vi "RemoveHandler.vi"(0 "Config in":T1, 5 "Server Index":i32, 7 "HandlerName":string, 11 "error in (no error)":errorcluster) -> (4 "Config out":T1, 15 "error out":errorcluster)   [LabVIEW 2017]
uses:
  <vilib>/WebServerConfig/Config.ctl
  <vilib>/WebServerConfig/Server.ctl
  <vilib>/WebServerConfig/Alias.ctl
  <vilib>/WebServerConfig/ErrorDocument.ctl
  <vilib>/WebServerConfig/Action.ctl
  <vilib>/WebServerConfig/Redirect.ctl
  <vilib>/WebServerConfig/Interface.ctl
  <vilib>/WebServerConfig/AddHandler.ctl
  <vilib>/WebServerConfig/SSL.ctl
  <vilib>/WebServerConfig/CustomLog.ctl
  <vilib>/WebServerConfig/LoadModule.ctl
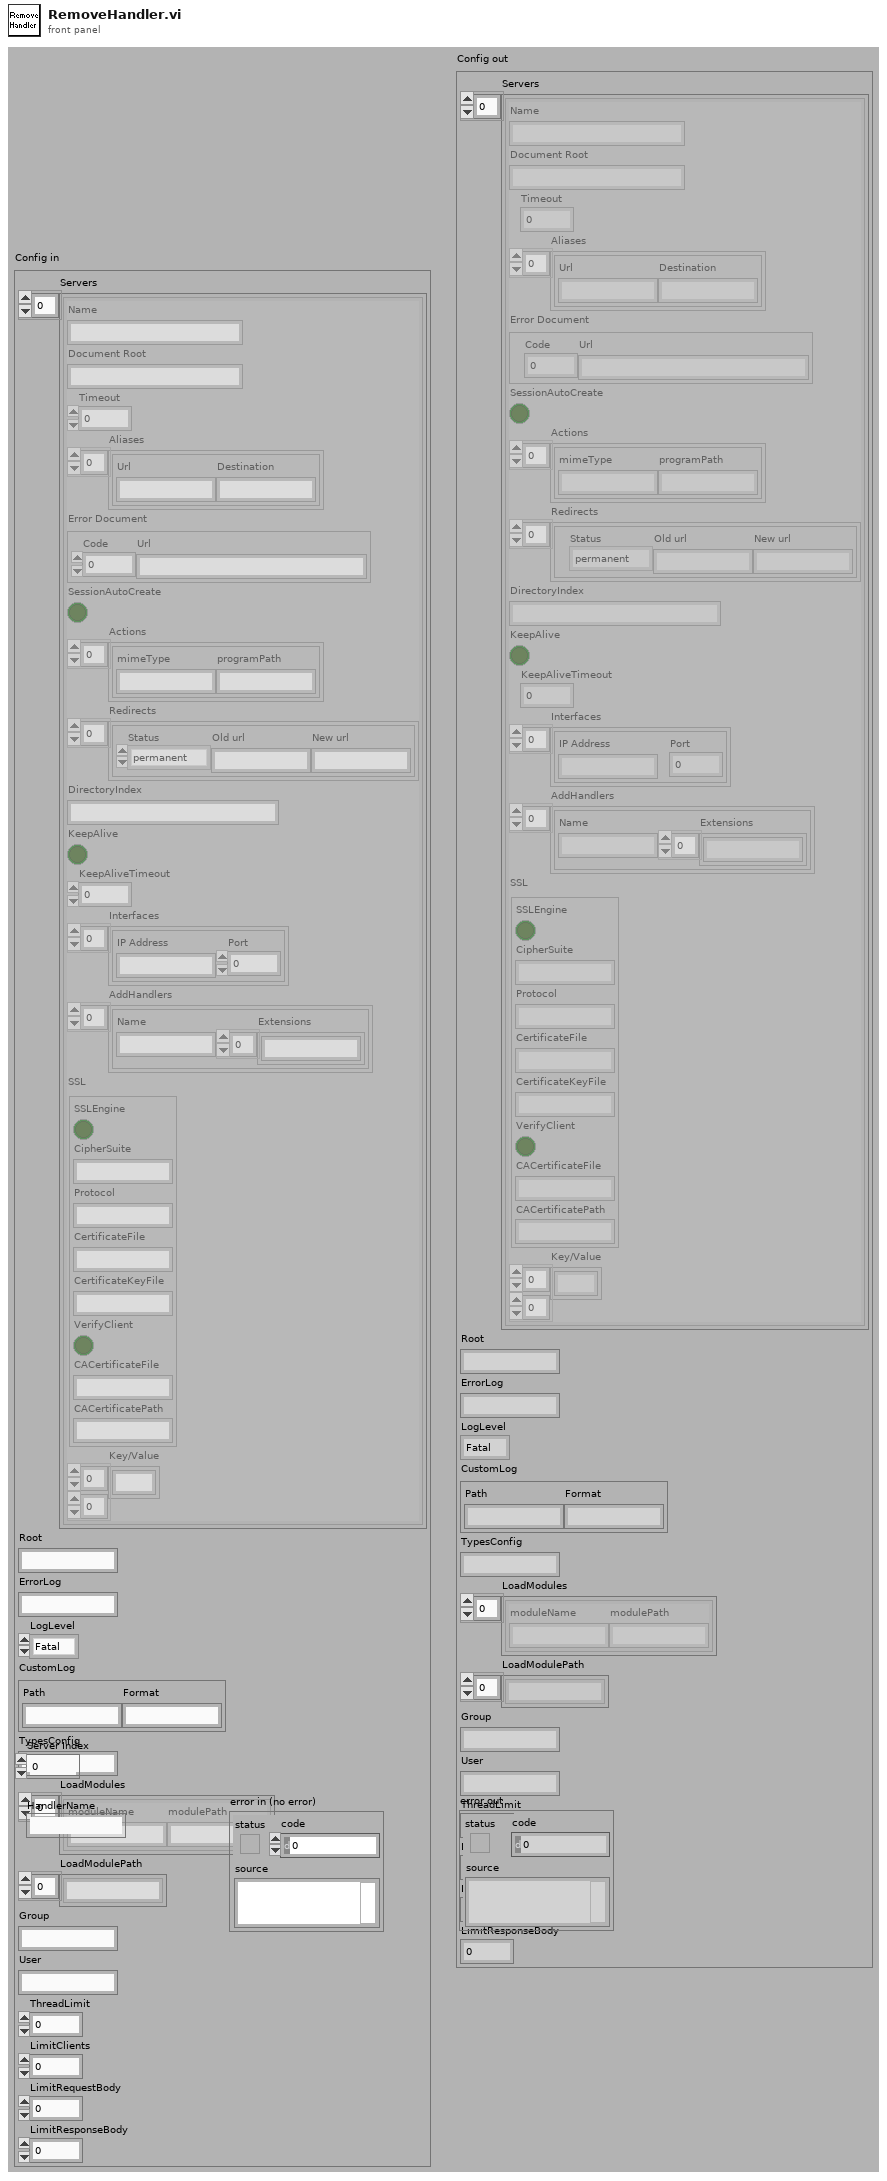
[diagram p1: front panel]
types:
  T1 = typedef "Config.ctl" = cluster{"Servers":T2[], "Root":string, "ErrorLog":string, "LogLevel":enum16{"Fatal", "Error", "Warn", "Info", "Debug", "5", "6", "7", "8", "Verbose"}, "CustomLog":T10, "TypesConfig":string, "LoadModules":T11[], "LoadModulePath":string[], "Group":string, "User":string, "ThreadLimit":u32, "LimitClients":u32, "LimitRequestBody":u32, "LimitResponseBody":u32}
  T2 = typedef "Server.ctl" = cluster{"Name":string, "Document Root":string, "Timeout":u32, "Aliases":T3[], "Error Document":T4, "SessionAutoCreate":bool, "Actions":T5[], "Redirects":T6[], "DirectoryIndex":string, "KeepAlive":bool, "KeepAliveTimeout":u32, "Interfaces":T7[], "AddHandlers":T8[], "SSL":T9, "Key/Value":string[][]}
  T3 = typedef "Alias.ctl" = cluster{"Url":string, "Destination":string}
  T4 = typedef "ErrorDocument.ctl" = cluster{"Code":u16, "Url":string}
  T5 = typedef "Action.ctl" = cluster{"mimeType":string, "programPath":string}
  T6 = typedef "Redirect.ctl" = cluster{"Status":enum16{"permanent", "temp", "seeother", "gone"}, "Old url":string, "New url":string}
  T7 = typedef "Interface.ctl" = cluster{"IP Address":string, "Port":u16}
  T8 = typedef "AddHandler.ctl" = cluster{"Name":string, "Extensions":string[]}
  T9 = typedef "SSL.ctl" = cluster{"SSLEngine":bool, "CipherSuite":string, "Protocol":string, "CertificateFile":string, "CertificateKeyFile":string, "VerifyClient":bool, "CACertificateFile":string, "CACertificatePath":string}
  T10 = typedef "CustomLog.ctl" = cluster{"Path":string, "Format":string}
  T11 = typedef "LoadModule.ctl" = cluster{"moduleName":string, "modulePath":string}
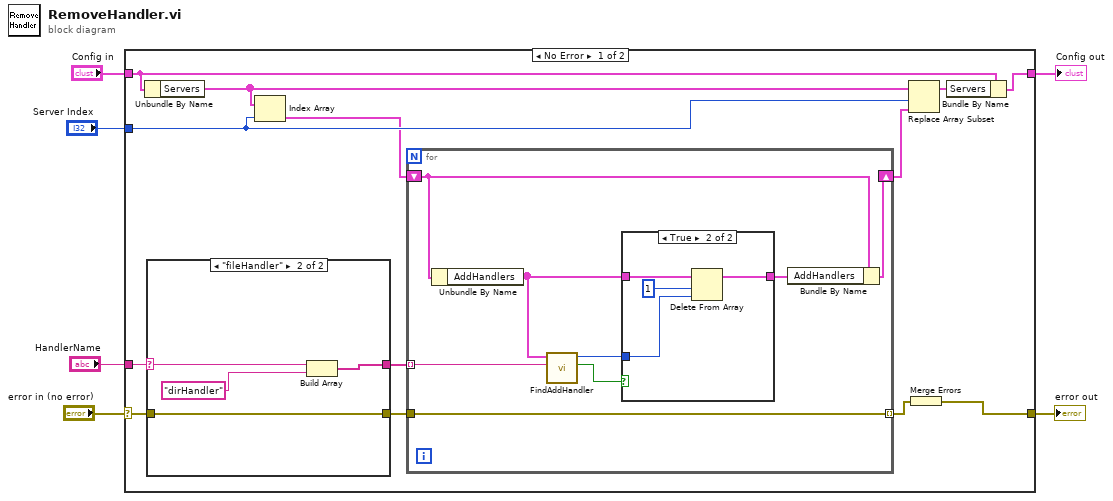
[diagram p0: block diagram]
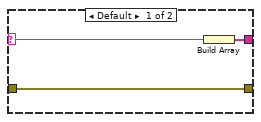
[diagram p3: hidden frame]
diagram:
  n1 = case shown="No Error" "error in (no error)" {
    selector: "error in (no error)" -> [w13 w41]
    tunnel: [w17 w40] -> w5
    tunnel: "Config in" -> [w18 w40]
    tunnel: [w11 w41] -> w3
    tunnel: "HandlerName" -> [w19 _]
    tunnel: "Server Index" -> [w14 _]
    frame No Error {
      n2 = Unbundle By Name(w18) -> ("Servers"=w15:T2[])
      n3 = case shown="\"fileHandler\"" w19 {
        selector: w19 -> [w33 w36]
        tunnel: w13 -> [w34 w39]
        tunnel: [w35 w38] -> w10
        tunnel: [w34 w39] -> w12
        frame Default {
          n4 = Build Array(w33) -> (w35:string[])
        }
        frame "fileHandler" {
          n5 = Build Array(w36, "dirHandler" ("Name")) -> (w38:string[])
        }
      }
      n6 = Index Array(array=w15, index=w14) -> (element=w9:T2)
      n7 = for {
        tunnel: w12 -> [w25]
        tunnel: w10 -> [w20] mode=indexing
        shift-right: [w26] -> w8
        shift-left: w9 -> [w27]
        tunnel: [w25] -> w7 mode=indexing
        n8 = Unbundle By Name(w27) -> ("AddHandlers"=w23:T8[])
        n9 = call <vilib>:"FindAddHandler.vi"("Name"=w20, "AddHandlers"=w23) -> ("Found"=w22:bool, "Index"=w21:i32)  [unwired: 8 in]
        n10 = case shown="True" w22 {
          tunnel: w23 -> [w28 w32]
          tunnel: [w28 w31] -> w24
          tunnel: w21 -> [_ w29]
          frame False {
          }
          frame True {
            n11 = Delete From Array(array=w32, length=1, index=w29) -> (array with subset deleted=w31:T8[])  [unwired: 1 out]
          }
        }
        n12 = Bundle By Name(cluster=w27, "AddHandlers"=w24) -> (w26:T2)
      }
      n13 = Replace Array Subset(array=w15, new element=w8, index=w14) -> (w16:T2[])
      n14 = Merge Errors(w7) -> (w11:errorcluster)
      n15 = Bundle By Name(cluster=w18, "Servers"=w16) -> (w17:T1)
    }
    frame Error {
    }
  }
  "Config out" <- w5
  "error out" <- w3
